vi "ExponentialLUTGenerator.vi"() -> ()   [LabVIEW 2018]
panel:
  in  "stop":bool
  out "String":string="-32768,-32768,-32768,-32767,-32767,-32766,-32766,-32765,-32764,-32763,-32762,-32760,-32759,-32757,-32756,-32754,-32752,-32750,-32748,-32745,-32743,-32740,-32738,-32735,-32732,-32729,-32726,-32722,-32719,-32715,-32712,-32708,-32704,-32700,-32696,-32691,-32687,-32682,-32678,-32673,-32668,-32663,-32658,-32652,-32647,-32641,-32636,-32630,-32624,-32618,-32612,-32605,-32599,-32592,-32586,-32579,-32572,-32565,-32558,-32550,-32543,-32535,-32528,-32520,-32512,-32504,-32496,-32487,-32479,-32470,-32462,-32453,-32444,-32435,-32426,-32416,-32407,-32397,-32388,-32378,-32368,-32358,-32348,-32337,-32327,-32316,-32306,-32295,-32284,-32273,-32262,-32250,-32239,-32227,-32216,-32204,-32192,-32180,-32168,-32155,-32143,-32130,-32118,-32105,-32092,-32079,-32066,-32052,-32039,-32025,-32012,-31998,-31984,-31970,-31956,-31941,-31927,-31912,-31898,-31883,-31868,-31853,-31838,-31822,-31807,-31791,-31776,-31760,-31744,-31728,-31712,-31695,-31679,-31662,-31646,-31629,-31612,-31595,-31578,-31560,-31543,-31525,-31508,-31490,-31472,-31454,-31436,-31417,-31399,-31380,-31362,-31343,-31324,-31305,-31286,-31266,-31247,-31227,-31208,-31188,-31168,-31148,-31128,-31107,-31087,-31066,-31046,-31025,-31004,-30983,-30962,-30940,-30919,-30897,-30876,-30854,-30832,-30810,-30788,-30765,-30743,-30720,-30698,-30675,-30652,-30629,-30606,-30582,-30559,-30535,-30512,-30488,-30464,-30440,-30416,-30391,-30367,-30342,-30318,-30293,-30268,-30243,-30218,-30192,-30167,-30141,-30116,-30090,-30064,-30038,-30012,-29985,-29959,-29932,-29906,-29879,-29852,-29825,-29798,-29770,-29743,-29715,-29688,-29660,-29632,-29604,-29576,-29547,-29519,-29490,-29462,-29433,-29404,-29375,-29346,-29316,-29287,-29257,-29228,-29198,-29168,-29138,-29108,-29077,-29047,-29016,-28986,-28955,-28924,-28893,-28862,-28830,-28799,-28767,-28736,-28704,-28672,-28640,-28608,-28575,-28543,-28510,-28478,-28445,-28412,-28379,-28346,-28312,-28279,-28245,-28212,-28178,-28144,-28110,-28076,-28041,-28007,-27972,-27938,-27903,-27868,-27833,-27798,-27762,-27727,-27691,-27656,-27620,-27584,-27548,-27512,-27475,-27439,-27402,-27366,-27329,-27292,-27255,-27218,-27180,-27143,-27105,-27068,-27030,-26992,-26954,-26916,-26877,-26839,-26800,-26762,-26723,-26684,-26645,-26606,-26566,-26527,-26487,-26448,-26408,-26368,-26328,-26288,-26247,-26207,-26166,-26126,-26085,-26044,-26003,-25962,-25920,-25879,-25837,-25796,-25754,-25712,-25670,-25628,-25585,-25543,-25500,-25458,-25415,-25372,-25329,-25286,-25242,-25199,-25155,-25112,-25068,-25024,-24980,-24936,-24891,-24847,-24802,-24758,-24713,-24668,-24623,-24578,-24532,-24487,-24441,-24396,-24350,-24304,-24258,-24212,-24165,-24119,-24072,-24026,-23979,-23932,-23885,-23838,-23790,-23743,-23695,-23648,-23600,-23552,-23504,-23456,-23407,-23359,-23310,-23262,-23213,-23164,-23115,-23066,-23016,-22967,-22917,-22868,-22818,-22768,-22718,-22668,-22617,-22567,-22516,-22466,-22415,-22364,-22313,-22262,-22210,-22159,-22107,-22056,-22004,-21952,-21900,-21848,-21795,-21743,-21690,-21638,-21585,-21532,-21479,-21426,-21372,-21319,-21265,-21212,-21158,-21104,-21050,-20996,-20941,-20887,-20832,-20778,-20723,-20668,-20613,-20558,-20502,-20447,-20391,-20336,-20280,-20224,-20168,-20112,-20055,-19999,-19942,-19886,-19829,-19772,-19715,-19658,-19600,-19543,-19485,-19428,-19370,-19312,-19254,-19196,-19137,-19079,-19020,-18962,-18903,-18844,-18785,-18726,-18666,-18607,-18547,-18488,-18428,-18368,-18308,-18248,-18187,-18127,-18066,-18006,-17945,-17884,-17823,-17762,-17700,-17639,-17577,-17516,-17454,-17392,-17330,-17268,-17205,-17143,-17080,-17018,-16955,-16892,-16829,-16766,-16702,-16639,-16575,-16512,-16448,-16384,-16320,-16256,-16191,-16127,-16062,-15998,-15933,-15868,-15803,-15738,-15672,-15607,-15541,-15476,-15410,-15344,-15278,-15212,-15145,-15079,-15012,-14946,-14879,-14812,-14745,-14678,-14610,-14543,-14475,-14408,-14340,-14272,-14204,-14136,-14067,-13999,-13930,-13862,-13793,-13724,-13655,-13586,-13516,-13447,-13377,-13308,-13238,-13168,-13098,-13028,-12957,-12887,-12816,-12746,-12675,-12604,-12533,-12462,-12390,-12319,-12247,-12176,-12104,-12032,-11960,-11888,-11815,-11743,-11670,-11598,-11525,-11452,-11379,-11306,-11232,-11159,-11085,-11012,-10938,-10864,-10790,-10716,-10641,-10567,-10492,-10418,-10343,-10268,-10193,-10118,-10042,-9967,-9891,-9816,-9740,-9664,-9588,-9512,-9435,-9359,-9282,-9206,-9129,-9052,-8975,-8898,-8820,-8743,-8665,-8588,-8510,-8432,-8354,-8276,-8197,-8119,-8040,-7962,-7883,-7804,-7725,-7646,-7566,-7487,-7407,-7328,-7248,-7168,-7088,-7008,-6927,-6847,-6766,-6686,-6605,-6524,-6443,-6362,-6280,-6199,-6117,-6036,-5954,-5872,-5790,-5708,-5625,-5543,-5460,-5378,-5295,-5212,-5129,-5046,-4962,-4879,-4795,-4712,-4628,-4544,-4460,-4376,-4291,-4207,-4122,-4038,-3953,-3868,-3783,-3698,-3612,-3527,-3441,-3356,-3270,-3184,-3098,-3012,-2925,-2839,-2752,-2666,-2579,-2492,-2405,-2318,-2230,-2143,-2055,-1968,-1880,-1792,-1704,-1616,-1527,-1439,-1350,-1262,-1173,-1084,-995,-906,-816,-727,-637,-548,-458,-368,-278,-188,-97,-7,84,174,265,356,447,538,630,721,813,904,996,1088,1180,1272,1365,1457,1550,1642,1735,1828,1921,2014,2108,2201,2295,2388,2482,2576,2670,2764,2859,2953,3048,3142,3237,3332,3427,3522,3618,3713,3809,3904,4000,4096,4192,4288,4385,4481,4578,4674,4771,4868,4965,5062,5160,5257,5355,5452,5550,5648,5746,5844,5943,6041,6140,6238,6337,6436,6535,6634,6734,6833,6933,7032,7132,7232,7332,7432,7533,7633,7734,7834,7935,8036,8137,8238,8340,8441,8543,8644,8746,8848,8950,9052,9155,9257,9360,9462,9565,9668,9771,9874,9978,10081,10185,10288,10392,10496,10600,10704,10809,10913,11018,11122,11227,11332,11437,11542,11648,11753,11859,11964,12070,12176,12282,12388,12495,12601,12708,12814,12921,13028,13135,13242,13350,13457,13565,13672,13780,13888,13996,14104,14213,14321,14430,14538,14647,14756,14865,14974,15084,15193,15303,15412,15522,15632,15742,15852,15963,16073,16184,16294,16405,16516,16627,16738,16850,16961,17073,17184,17296,17408,17520,17632,17745,17857,17970,18082,18195,18308,18421,18534,18648,18761,18875,18988,19102,19216,19330,19444,19559,19673,19788,19902,20017,20132,20247,20362,20478,20593,20709,20824,20940,21056,21172,21288,21405,21521,21638,21754,21871,21988,22105,22222,22340,22457,22575,22692,22810,22928,23046,23164,23283,23401,23520,23638,23757,23876,23995,24114,24234,24353,24473,24592,24712,24832,24952,25072,25193,25313,25434,25554,25675,25796,25917,26038,26160,26281,26403,26524,26646,26768,26890,27012,27135,27257,27380,27502,27625,27748,27871,27994,28118,28241,28365,28488,28612,28736,28860,28984,29109,29233,29358,29482,29607,29732,29857,29982,30108,30233,30359,30484,30610,30736,30862,30988,31115,31241,31368,31494,31621,31748,31875,32002,32130,32257,32385,32512,32640,"
  in  "MIN":dbl=32768.0
  in  "MAX":dbl=65536.0
  in  "Steap":dbl=2.0
  out "Waveform Graph":dbl[](graph)=[-32768.0, -32767.9375, -32767.75, -32767.4375, -32767.0, -32766.4375, -32765.75, -32764.9375, -32764.0, -32762.9375, -32761.75, -32760.4375, -32759.0, -32757.4375, -32755.75, -32753.9375, -32752.0, -32749.9375, -32747.75, -32745.4375, -32743.0, -32740.4375, -32737.75, -32734.9375, -32732.0, -32728.9375, -32725.75, -32722.4375, -32719.0, -32715.4375, -32711.75, -32707.9375, -32704.0, -32699.9375, -32695.75, -32691.4375, -32687.0, -32682.4375, -32677.75, -32672.9375, -32668.0, -32662.9375, -32657.75, -32652.4375, -32647.0, -32641.4375, -32635.75, -32629.9375, -32624.0, -32617.9375, -32611.75, -32605.4375, -32599.0, -32592.4375, -32585.75, -32578.9375, -32572.0, -32564.9375, -32557.75, -32550.4375, -32543.0, -32535.4375, -32527.75, -32519.9375, -32512.0, -32503.9375, -32495.75, -32487.4375, -32479.0, -32470.4375, -32461.75, -32452.9375, -32444.0, -32434.9375, -32425.75, -32416.4375, -32407.0, -32397.4375, -32387.75, -32377.9375, -32368.0, -32357.9375, -32347.75, -32337.4375, -32327.0, -32316.4375, -32305.75, -32294.9375, -32284.0, -32272.9375, -32261.75, -32250.4375, -32239.0, -32227.4375, -32215.75, -32203.9375, -32192.0, -32179.9375, -32167.75, -32155.4375, -32143.0, -32130.4375, -32117.75, -32104.9375, -32092.0, -32078.9375, -32065.75, -32052.4375, -32039.0, -32025.4375, -32011.75, -31997.9375, -31984.0, -31969.9375, -31955.75, -31941.4375, -31927.0, -31912.4375, -31897.75, -31882.9375, -31868.0, -31852.9375, -31837.75, -31822.4375, -31807.0, -31791.4375, -31775.75, -31759.9375, -31744.0, -31727.9375, -31711.75, -31695.4375, -31679.0, -31662.4375, -31645.75, -31628.9375, -31612.0, -31594.9375, -31577.75, -31560.4375, -31543.0, -31525.4375, -31507.75, -31489.9375, -31472.0, -31453.9375, -31435.75, -31417.4375, -31399.0, -31380.4375, -31361.75, -31342.9375, -31324.0, -31304.9375, -31285.75, -31266.4375, -31247.0, -31227.4375, -31207.75, -31187.9375, -31168.0, -31147.9375, -31127.75, -31107.4375, -31087.0, -31066.4375, -31045.75, -31024.9375, -31004.0, -30982.9375, -30961.75, -30940.4375, -30919.0, -30897.4375, -30875.75, -30853.9375, -30832.0, -30809.9375, -30787.75, -30765.4375, -30743.0, -30720.4375, -30697.75, -30674.9375, -30652.0, -30628.9375, -30605.75, -30582.4375, -30559.0, -30535.4375, -30511.75, -30487.9375, -30464.0, -30439.9375, -30415.75, -30391.4375, -30367.0, -30342.4375, -30317.75, -30292.9375, -30268.0, -30242.9375, -30217.75, -30192.4375, -30167.0, -30141.4375, -30115.75, -30089.9375, -30064.0, -30037.9375, -30011.75, -29985.4375, -29959.0, -29932.4375, -29905.75, -29878.9375, -29852.0, -29824.9375, -29797.75, -29770.4375, -29743.0, -29715.4375, -29687.75, -29659.9375, -29632.0, -29603.9375, -29575.75, -29547.4375, -29519.0, -29490.4375, -29461.75, -29432.9375, -29404.0, -29374.9375, -29345.75, -29316.4375, -29287.0, -29257.4375, -29227.75, -29197.9375, -29168.0, -29137.9375, -29107.75, -29077.4375, -29047.0, -29016.4375, -28985.75, -28954.9375, -28924.0, -28892.9375, -28861.75, -28830.4375, -28799.0, -28767.4375, -28735.75, -28703.9375, -28672.0, -28639.9375, -28607.75, -28575.4375, -28543.0, -28510.4375, -28477.75, -28444.9375, -28412.0, -28378.9375, -28345.75, -28312.4375, -28279.0, -28245.4375, -28211.75, -28177.9375, -28144.0, -28109.9375, -28075.75, -28041.4375, -28007.0, -27972.4375, -27937.75, -27902.9375, -27868.0, -27832.9375, -27797.75, -27762.4375, -27727.0, -27691.4375, -27655.75, -27619.9375, -27584.0, -27547.9375, -27511.75, -27475.4375, -27439.0, -27402.4375, -27365.75, -27328.9375, -27292.0, -27254.9375, -27217.75, -27180.4375, -27143.0, -27105.4375, -27067.75, -27029.9375, -26992.0, -26953.9375, -26915.75, -26877.4375, -26839.0, -26800.4375, -26761.75, -26722.9375, -26684.0, -26644.9375, -26605.75, -26566.4375, -26527.0, -26487.4375, -26447.75, -26407.9375, -26368.0, -26327.9375, -26287.75, -26247.4375, -26207.0, -26166.4375, -26125.75, -26084.9375, -26044.0, -26002.9375, -25961.75, -25920.4375, -25879.0, -25837.4375, -25795.75, -25753.9375, -25712.0, -25669.9375, -25627.75, -25585.4375, -25543.0, -25500.4375, -25457.75, -25414.9375, -25372.0, -25328.9375, -25285.75, -25242.4375, -25199.0, -25155.4375, -25111.75, -25067.9375, -25024.0, -24979.9375, -24935.75, -24891.4375, -24847.0, -24802.4375, -24757.75, -24712.9375, -24668.0, -24622.9375, -24577.75, -24532.4375, -24487.0, -24441.4375, -24395.75, -24349.9375, -24304.0, -24257.9375, -24211.75, -24165.4375, -24119.0, -24072.4375, -24025.75, -23978.9375, -23932.0, -23884.9375, -23837.75, -23790.4375, -23743.0, -23695.4375, -23647.75, -23599.9375, -23552.0, -23503.9375, -23455.75, -23407.4375, -23359.0, -23310.4375, -23261.75, -23212.9375, -23164.0, -23114.9375, -23065.75, -23016.4375, -22967.0, -22917.4375, -22867.75, -22817.9375, -22768.0, -22717.9375, -22667.75, -22617.4375, -22567.0, -22516.4375, -22465.75, -22414.9375, -22364.0, -22312.9375, -22261.75, -22210.4375, -22159.0, -22107.4375, -22055.75, -22003.9375, -21952.0, -21899.9375, -21847.75, -21795.4375, -21743.0, -21690.4375, -21637.75, -21584.9375, -21532.0, -21478.9375, -21425.75, -21372.4375, -21319.0, -21265.4375, -21211.75, -21157.9375, -21104.0, -21049.9375, -20995.75, -20941.4375, -20887.0, -20832.4375, -20777.75, -20722.9375, -20668.0, -20612.9375, -20557.75, -20502.4375, -20447.0, -20391.4375, -20335.75, -20279.9375, -20224.0, -20167.9375, -20111.75, -20055.4375, -19999.0, -19942.4375, -19885.75, -19828.9375, -19772.0, -19714.9375, -19657.75, -19600.4375, -19543.0, -19485.4375, -19427.75, -19369.9375, -19312.0, -19253.9375, -19195.75, -19137.4375, -19079.0, -19020.4375, -18961.75, -18902.9375, -18844.0, -18784.9375, -18725.75, -18666.4375, -18607.0, -18547.4375, -18487.75, -18427.9375, -18368.0, -18307.9375, -18247.75, -18187.4375, -18127.0, -18066.4375, -18005.75, -17944.9375, -17884.0, -17822.9375, -17761.75, -17700.4375, -17639.0, -17577.4375, -17515.75, -17453.9375, -17392.0, -17329.9375, -17267.75, -17205.4375, -17143.0, -17080.4375, -17017.75, -16954.9375, -16892.0, -16828.9375, -16765.75, -16702.4375, -16639.0, -16575.4375, -16511.75, -16447.9375, -16384.0, -16319.9375, -16255.75, -16191.4375, -16127.0, -16062.4375, -15997.75, -15932.9375, -15868.0, -15802.9375, -15737.75, -15672.4375, -15607.0, -15541.4375, -15475.75, -15409.9375, -15344.0, -15277.9375, -15211.75, -15145.4375, -15079.0, -15012.4375, -14945.75, -14878.9375, -14812.0, -14744.9375, -14677.75, -14610.4375, -14543.0, -14475.4375, -14407.75, -14339.9375, -14272.0, -14203.9375, -14135.75, -14067.4375, -13999.0, -13930.4375, -13861.75, -13792.9375, -13724.0, -13654.9375, -13585.75, -13516.4375, -13447.0, -13377.4375, -13307.75, -13237.9375, -13168.0, -13097.9375, -13027.75, -12957.4375, -12887.0, -12816.4375, -12745.75, -12674.9375, -12604.0, -12532.9375, -12461.75, -12390.4375, -12319.0, -12247.4375, -12175.75, -12103.9375, -12032.0, -11959.9375, -11887.75, -11815.4375, -11743.0, -11670.4375, -11597.75, -11524.9375, -11452.0, -11378.9375, -11305.75, -11232.4375, -11159.0, -11085.4375, -11011.75, -10937.9375, -10864.0, -10789.9375, -10715.75, -10641.4375, -10567.0, -10492.4375, -10417.75, -10342.9375, -10268.0, -10192.9375, -10117.75, -10042.4375, -9967.0, -9891.4375, -9815.75, -9739.9375, -9664.0, -9587.9375, -9511.75, -9435.4375, -9359.0, -9282.4375, -9205.75, -9128.9375, -9052.0, -8974.9375, -8897.75, -8820.4375, -8743.0, -8665.4375, -8587.75, -8509.9375, -8432.0, -8353.9375, -8275.75, -8197.4375, -8119.0, -8040.4375, -7961.75, -7882.9375, -7804.0, -7724.9375, -7645.75, -7566.4375, -7487.0, -7407.4375, -7327.75, -7247.9375, -7168.0, -7087.9375, -7007.75, -6927.4375, -6847.0, -6766.4375, -6685.75, -6604.9375, -6524.0, -6442.9375, -6361.75, -6280.4375, -6199.0, -6117.4375, -6035.75, -5953.9375, -5872.0, -5789.9375, -5707.75, -5625.4375, -5543.0, -5460.4375, -5377.75, -5294.9375, -5212.0, -5128.9375, -5045.75, -4962.4375, -4879.0, -4795.4375, -4711.75, -4627.9375, -4544.0, -4459.9375, -4375.75, -4291.4375, -4207.0, -4122.4375, -4037.75, -3952.9375, -3868.0, -3782.9375, -3697.75, -3612.4375, -3527.0, -3441.4375, -3355.75, -3269.9375, -3184.0, -3097.9375, -3011.75, -2925.4375, -2839.0, -2752.4375, -2665.75, -2578.9375, -2492.0, -2404.9375, -2317.75, -2230.4375, -2143.0, -2055.4375, -1967.75, -1879.9375, -1792.0, -1703.9375, -1615.75, -1527.4375, -1439.0, -1350.4375, -1261.75, -1172.9375, -1084.0, -994.9375, -905.75, -816.4375, -727.0, -637.4375, -547.75, -457.9375, -368.0, -277.9375, -187.75, -97.4375, -7.0, 83.5625, 174.25, 265.0625, 356.0, 447.0625, 538.25, 629.5625, 721.0, 812.5625, 904.25, 996.0625, 1088.0, 1180.0625, 1272.25, 1364.5625, 1457.0, 1549.5625, 1642.25, 1735.0625, 1828.0, 1921.0625, 2014.25, 2107.5625, 2201.0, 2294.5625, 2388.25, 2482.0625, 2576.0, 2670.0625, 2764.25, 2858.5625, 2953.0, 3047.5625, 3142.25, 3237.0625, 3332.0, 3427.0625, 3522.25, 3617.5625, 3713.0, 3808.5625, 3904.25, 4000.0625, 4096.0, 4192.0625, 4288.25, 4384.5625, 4481.0, 4577.5625, 4674.25, 4771.0625, 4868.0, 4965.0625, 5062.25, 5159.5625, 5257.0, 5354.5625, 5452.25, 5550.0625, 5648.0, 5746.0625, 5844.25, 5942.5625, 6041.0, 6139.5625, 6238.25, 6337.0625, 6436.0, 6535.0625, 6634.25, 6733.5625, 6833.0, 6932.5625, 7032.25, 7132.0625, 7232.0, 7332.0625, 7432.25, 7532.5625, 7633.0, 7733.5625, 7834.25, 7935.0625, 8036.0, 8137.0625, 8238.25, 8339.5625, 8441.0, 8542.5625, 8644.25, 8746.0625, 8848.0, 8950.0625, 9052.25, 9154.5625, 9257.0, 9359.5625, 9462.25, 9565.0625, 9668.0, 9771.0625, 9874.25, 9977.5625, 10081.0, 10184.5625, 10288.25, 10392.0625, 10496.0, 10600.0625, 10704.25, 10808.5625, 10913.0, 11017.5625, 11122.25, 11227.0625, 11332.0, 11437.0625, 11542.25, 11647.5625, 11753.0, 11858.5625, 11964.25, 12070.0625, 12176.0, 12282.0625, 12388.25, 12494.5625, 12601.0, 12707.5625, 12814.25, 12921.0625, 13028.0, 13135.0625, 13242.25, 13349.5625, 13457.0, 13564.5625, 13672.25, 13780.0625, 13888.0, 13996.0625, 14104.25, 14212.5625, 14321.0, 14429.5625, 14538.25, 14647.0625, 14756.0, 14865.0625, 14974.25, 15083.5625, 15193.0, 15302.5625, 15412.25, 15522.0625, 15632.0, 15742.0625, 15852.25, 15962.5625, 16073.0, 16183.5625, 16294.25, 16405.0625, 16516.0, 16627.0625, 16738.25, 16849.5625, 16961.0, 17072.5625, 17184.25, 17296.0625, 17408.0, 17520.0625, 17632.25, 17744.5625, 17857.0, 17969.5625, 18082.25, 18195.0625, 18308.0, 18421.0625, 18534.25, 18647.5625, 18761.0, 18874.5625, 18988.25, 19102.0625, 19216.0, 19330.0625, 19444.25, 19558.5625, 19673.0, 19787.5625, 19902.25, 20017.0625, 20132.0, 20247.0625, 20362.25, 20477.5625, 20593.0, 20708.5625, 20824.25, 20940.0625, 21056.0, 21172.0625, 21288.25, 21404.5625, 21521.0, 21637.5625, 21754.25, 21871.0625, 21988.0, 22105.0625, 22222.25, 22339.5625, 22457.0, 22574.5625, 22692.25, 22810.0625, 22928.0, 23046.0625, 23164.25, 23282.5625, 23401.0, 23519.5625, 23638.25, 23757.0625, 23876.0, 23995.0625, 24114.25, 24233.5625, 24353.0, 24472.5625, 24592.25, 24712.0625, 24832.0, 24952.0625, 25072.25, 25192.5625, 25313.0, 25433.5625, 25554.25, 25675.0625, 25796.0, 25917.0625, 26038.25, 26159.5625, 26281.0, 26402.5625, 26524.25, 26646.0625, 26768.0, 26890.0625, 27012.25, 27134.5625, 27257.0, 27379.5625, 27502.25, 27625.0625, 27748.0, 27871.0625, 27994.25, 28117.5625, 28241.0, 28364.5625, 28488.25, 28612.0625, 28736.0, 28860.0625, 28984.25, 29108.5625, 29233.0, 29357.5625, 29482.25, 29607.0625, 29732.0, 29857.0625, 29982.25, 30107.5625, 30233.0, 30358.5625, 30484.25, 30610.0625, 30736.0, 30862.0625, 30988.25, 31114.5625, 31241.0, 31367.5625, 31494.25, 31621.0625, 31748.0, 31875.0625, 32002.25, 32129.5625, 32257.0, 32384.5625, 32512.25, 32640.0625]
  in  "Length":i32=1024
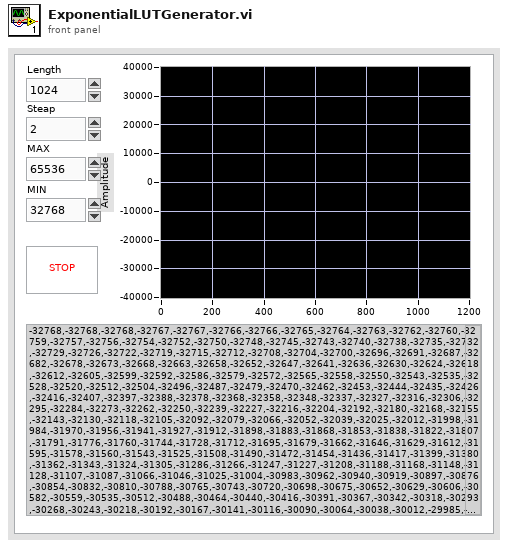
[diagram p1: front panel]
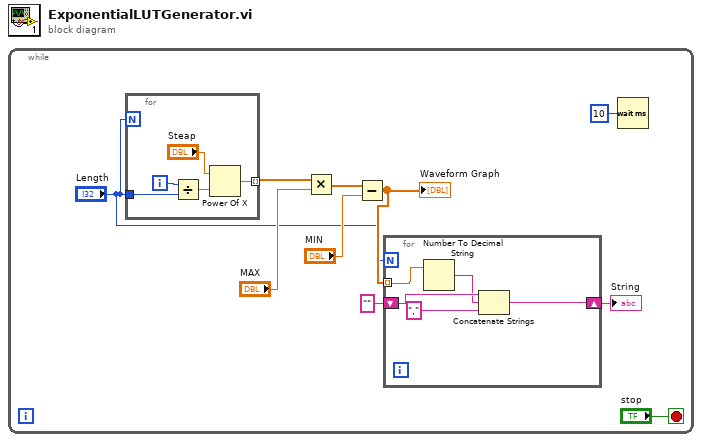
[diagram p0: block diagram]
diagram:
  n1 = while {
    stop <- "stop" stop-if-true
    n2 = for {
      N: "Length" -> [_]
      tunnel: "Length" -> [w20]
      tunnel: [w17] -> w10 mode=indexing
      i -> [w19]
      n3 = Divide(x=w19, y=w20) -> (x/y=w18:dbl)
      n4 = Power Of X(1:w18, 2:"Steap") -> (0:w17:dbl)
    }
    n5 = Multiply(x=w10, y="MAX") -> (x*y=w9:dbl[])
    n6 = Subtract(x=w9, y="MIN") -> (x-y=w6:dbl[])
    "Waveform Graph" <- w6
    n7 = for {
      N: "Length" -> [_]
      shift-right: [w14] -> w5
      shift-left: "" -> [w13]
      tunnel: w6 -> [w11] mode=indexing
      n8 = Number To Decimal String(number=w11) -> (decimal integer string=w12:string)  [unwired: 1 in]
      n9 = Concatenate Strings(w13, w12, "," ("string")) -> (w14:string)
    }
    "String" <- w5
    n10 = Wait (ms)(milliseconds to wait=u32 10) -> ()  [unwired: 1 out]
  }
